vi "XY Graph.vi"() -> ()   [LabVIEW 2025]
panel:
  out "XY Graph 3":cluster{dbl[], dbl[]}[](graph)
  out "XY Graph 2":cluster{timestamp[], dbl[]}(graph)
  out "XY Graph":cluster{dbl[], dbl[]}(graph)
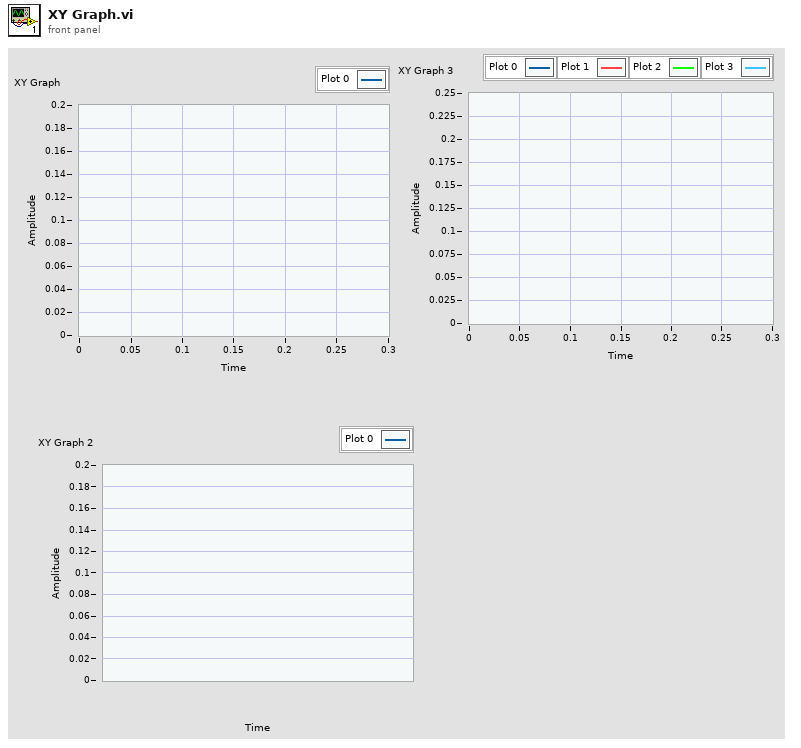
[diagram p1: front panel]
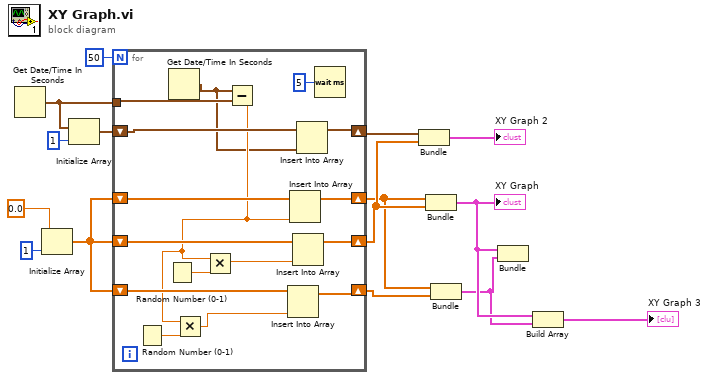
[diagram p0: block diagram]
diagram:
  n1 = Get Date/Time In Seconds() -> (seconds since 1Jan1904=w12:timestamp)
  n2 = Initialize Array(0.0 ("element"), 1 ("dimension size")) -> (w13:dbl[])
  n3 = Initialize Array(w12, 1 ("dimension size")) -> (w10:timestamp[])
  n4 = for {
    N: 50 -> [_]
    shift-right: [w28] -> w4
    shift-left: w13 -> [w27]
    shift-right: [w18] -> w5
    shift-left: w13 -> [w21]
    shift-right: [w24] -> w7
    shift-left: w13 -> [w25]
    tunnel: w12 -> [w31]
    shift-right: [w29] -> w8
    shift-left: w10 -> [w30]
    n5 = Random Number (0-1)() -> (number: 0 to 1=w22:dbl)
    n6 = Random Number (0-1)() -> (number: 0 to 1=w26:dbl)
    n7 = Get Date/Time In Seconds() -> (seconds since 1Jan1904=w16:timestamp)
    n8 = Subtract(x=w16, y=w31) -> (x-y=w20:dbl)
    n9 = Multiply(x=w20, y=w22) -> (x*y=w19:dbl)
    n10 = Multiply(x=w20, y=w26) -> (x*y=w23:dbl)
    n11 = Insert Into Array(array=w21, new element=w19) -> (w18:dbl[])  [unwired: 1 in]
    n12 = Insert Into Array(array=w27, new element=w20) -> (w28:dbl[])  [unwired: 1 in]
    n13 = Insert Into Array(array=w25, new element=w23) -> (w24:dbl[])  [unwired: 1 in]
    n14 = Insert Into Array(array=w30, new element=w16) -> (w29:timestamp[])  [unwired: 1 in]
    n15 = Wait (ms)(milliseconds to wait=u32 5) -> ()  [unwired: 1 out]
  }
  n16 = Bundle(w8, w7) -> (→"XY Graph 2":cluster{timestamp[], dbl[]})  [unwired: 1 in]
  n17 = Bundle(w4, w7) -> (w3:cluster{dbl[], dbl[]})  [unwired: 1 in]
  "XY Graph" <- w3
  n18 = Bundle(w4, w5) -> (w2:cluster{dbl[], dbl[]})  [unwired: 1 in]
  n19 = Bundle(w3, w2) -> ()  [unwired: 1 in, 1 out]
  n20 = Build Array(w3, w2) -> (→"XY Graph 3":cluster{dbl[], dbl[]}[])
